vi "settle timer start.vi"(2 "in settle band":bool, 7 "Control Parameters":T1={"Setpoint"=50.0, "Control Bandwidth"=4.0, "Integral Time"=30.0, "Int\nON"=TRUE, "Derivative Tme"=0.5, "Der\nON"=TRUE, "Settle Bandwidth"=1.0, "Settle Time"=200.0} {"Settle Time" step=1.0; "Settle Bandwidth" step=0.01; "Derivative Tme" step=0.01; "Integral Time" step=1.0; "Control Bandwidth" step=0.1; "Setpoint" step=0.1}, 9 "reset":bool, 11 "delta t":dbl format="%.2f") -> (8 "time in settle band":dbl format="%.2f", 15 "settled":bool)   [LabVIEW 2019]
doc: "Subvi check to see if temperature is settled over set period of time true if settle time is greater than set time \n\nJuan Gamez \nP3600\nCSUSB"
uses:
  typedefs/PID control parameters.ctl
panel:
  # "settle timer"
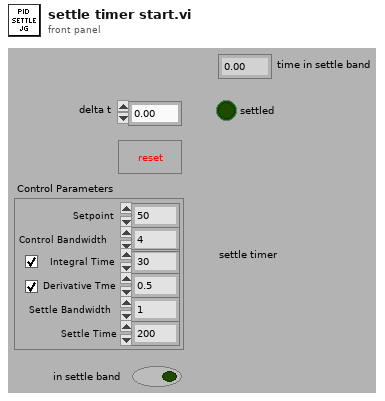
[diagram p1: front panel]
types:
  T1 = typedef "PID control parameters.ctl" = cluster{"Setpoint":dbl, "Control Bandwidth":dbl, "Integral Time":dbl, "Int\nON":bool, "Derivative Tme":dbl, "Der\nON":bool, "Settle Bandwidth":dbl, "Settle Time":dbl}
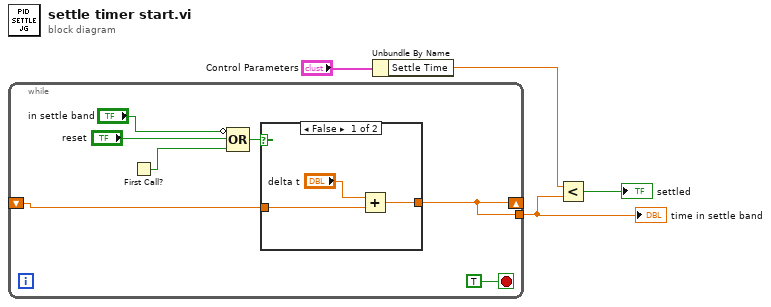
[diagram p0: block diagram]
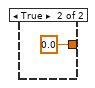
[diagram p2: hidden frame]
diagram:
  n1 = while {
    shift-right: [w6] -> _
    shift-left: _ -> [w7]
    tunnel: [w6] -> w3
    stop <- TRUE stop-if-true
    n2 = First Call?() -> (First Call?: T/F=w11:bool)
    n3 = Compound Arithmetic op=OR(invert "in settle band", "reset", w11) -> (w8:bool)
    n4 = case shown="False" w8 {
      tunnel: [w13 0.0] -> w6
      tunnel: w7 -> [w12 _]
      frame False {
        n5 = Add(x="delta t", y=w12) -> (x+y=w13:dbl)
      }
      frame True {
      }
    }
  }
  "time in settle band" <- w3
  n6 = Unbundle By Name("Control Parameters") -> ("Settle Time"=w2:dbl)
  n7 = Less?(x=w2, y=w3) -> (x < y?=→"settled":bool)
